vi "NCC DLL Test.vi"() -> ()   [LabVIEW 2016]
uses:
  Microscope Control/Microscope Modules/Wide Field Drift Correction/WFDC DLL and Testing/Visual Studio NCC Max Shift DLL/x64/Release/VSmaxShiftNCC.dll
panel:
  out "Time (s)":dbl
  out "Intensity Graph":dbl[][](graph)
  out "theResult":dbl[][](array[numeric])
  in  "Test Image 02":path=path "C:/Users/George Sirinakis/Documents/Microscope Control/Microscope Modules/Wide Field Drift Correction/WFDC DLL and Testing/Egg Chamber Test Data/Stack02/Color02/Color02_00001.tif"
  in  "Test Image 01":path=path "C:/Users/George Sirinakis/Documents/Microscope Control/Microscope Modules/Wide Field Drift Correction/WFDC DLL and Testing/Egg Chamber Test Data/Stack02/Color02/Color02_00007.tif"
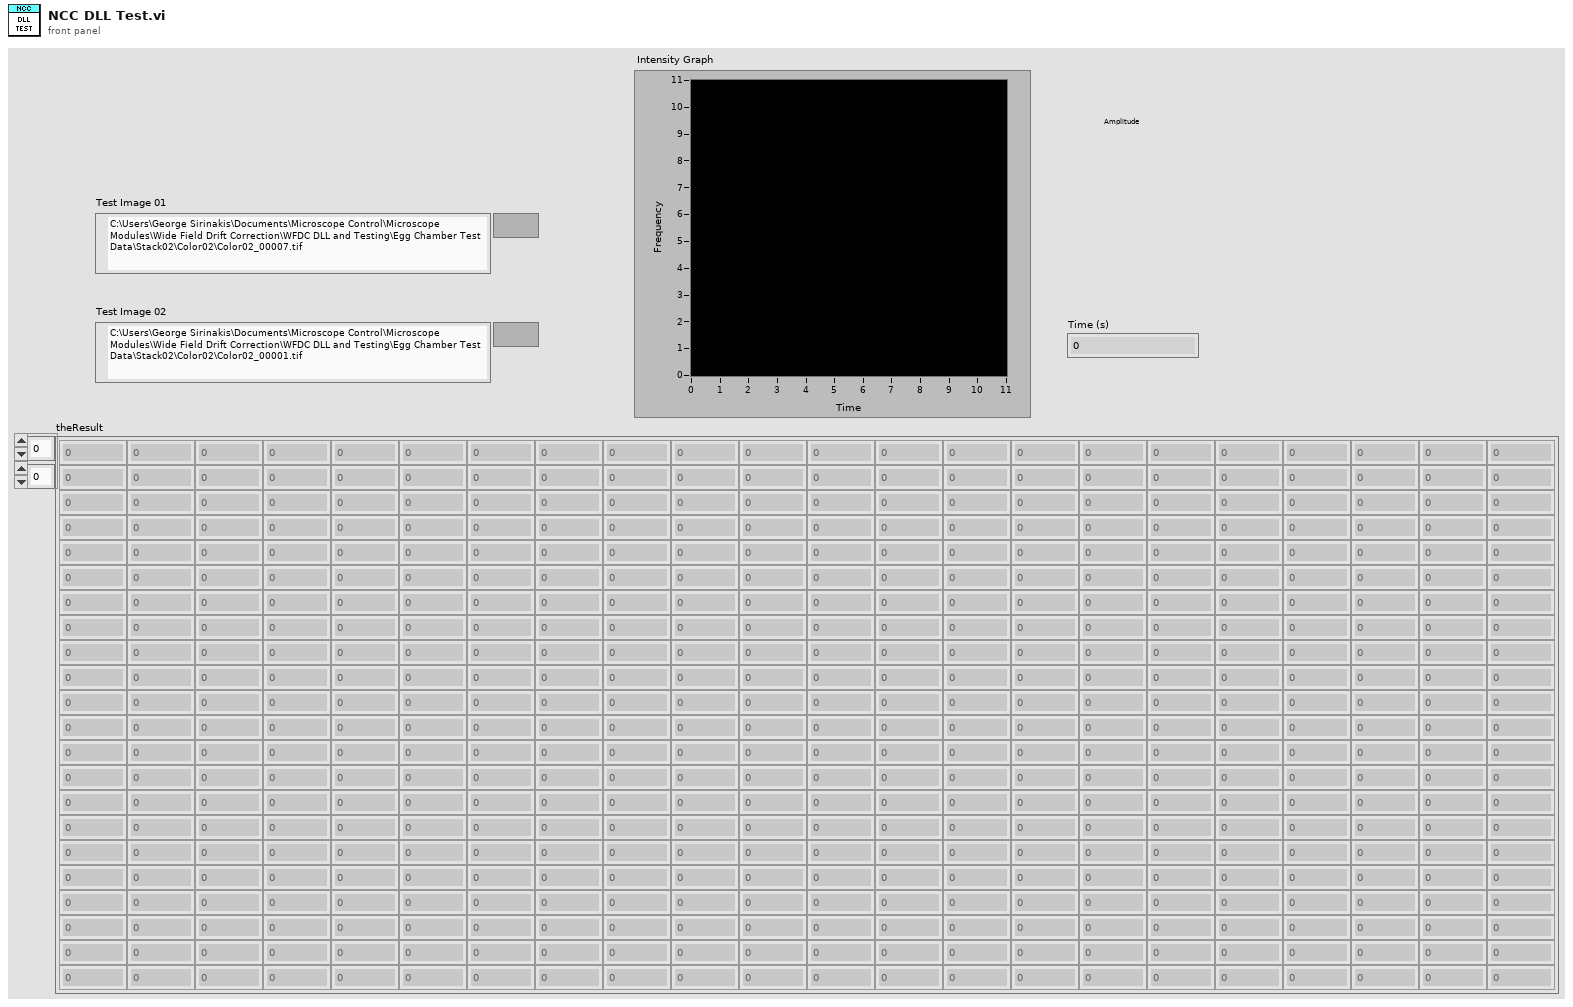
[diagram p1: front panel]
types:
  T1 = typedef "Image Type" = u32
  T2 = typedef "IMAQ Image.ctl" = refnum<image>
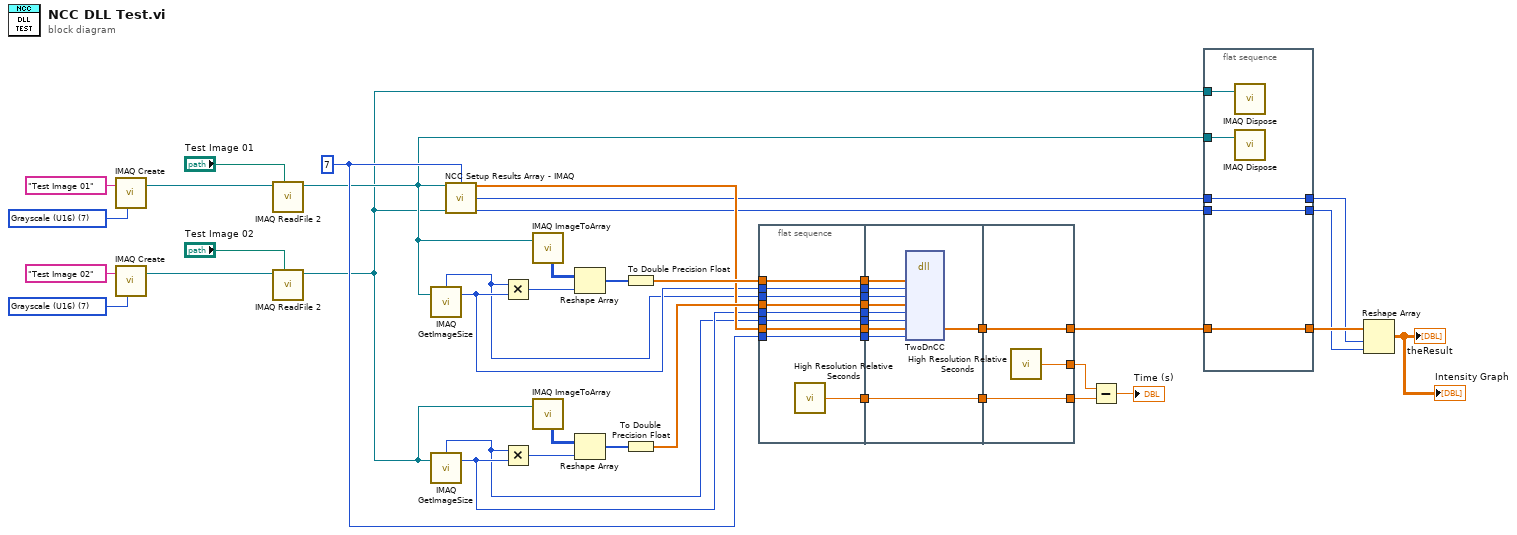
[diagram p0: block diagram]
diagram:
  w42 = T1 7 items=["Grayscale (U8)", "Grayscale (I16)", "Grayscale (SGL)", "Complex (CSG)", "RGB (U32)", "HSL (U32)", "RGB (U64)", "Grayscale (U16)"] ("Image Type")
  w43 = T1 7 items=["Grayscale (U8)", "Grayscale (I16)", "Grayscale (SGL)", "Complex (CSG)", "RGB (U32)", "HSL (U32)", "RGB (U64)", "Grayscale (U16)"] ("Image Type")
  w28 = 7 ("Half Shift")
  n1 = call "IMAQ Create"("Image Name"="Test Image 01", "Image Type"=w43) -> ("New Image"=w41:T2)  [unwired: 3 in, 1 out]
  n2 = call "IMAQ Create"("Image Name"="Test Image 02", "Image Type"=w42) -> ("New Image"=w40:T2)  [unwired: 3 in, 1 out]
  n3 = call "IMAQ ReadFile 2"("File Path"="Test Image 01", "Image"=w41) -> ("Image Out"=w22:T2)  [unwired: 5 in, 4 out]
  n4 = call "IMAQ ReadFile 2"("File Path"="Test Image 02", "Image"=w40) -> ("Image Out"=w21:T2)  [unwired: 5 in, 4 out]
  n5 = call "IMAQ GetImageSize"("Image"=w22) -> ("Y Resolution"=w25:i32, "X Resolution"=w24:i32)  [unwired: 3 in, 1 out]
  n6 = call "IMAQ GetImageSize"("Image"=w21) -> ("Y Resolution"=w27:i32, "X Resolution"=w26:i32)  [unwired: 3 in, 1 out]
  n7 = call "NCC Setup Results Array - IMAQ.vi"("Image Ref 01"=w22, "Half Shift"=w28, "Image Ref 02"=w21) -> ("NCC Results Array"=w29:dbl[], "Result Rows"=w20:i32, "Result Columns"=w19:i32)  [unwired: 10 in]
  n8 = Multiply(x=w24, y=w25) -> (x*y=w35:i32)
  n9 = Multiply(x=w26, y=w27) -> (x*y=w36:i32)
  n10 = call "IMAQ ImageToArray"("Image"=w22) -> ("Image Pixels (U16)"=w34:u16[][])  [unwired: 3 in, 4 out]
  n11 = call "IMAQ ImageToArray"("Image"=w21) -> ("Image Pixels (U16)"=w37:u16[][])  [unwired: 3 in, 4 out]
  n12 = Reshape Array(w34, w35) -> (w33:u16[])
  n13 = Reshape Array(w37, w36) -> (w32:u16[])
  n14 = To Double Precision Float(number=w33) -> (double precision float=w31:dbl[])
  n15 = To Double Precision Float(number=w32) -> (double precision float=w30:dbl[])
  n16 = flat-sequence {
    tunnel: w24 -> [w47]
    tunnel: w25 -> [w48]
    tunnel: w26 -> [w49]
    tunnel: w27 -> [w50]
    tunnel: w28 -> [w51]
    tunnel: w29 -> [w52]
    tunnel: w30 -> [w53]
    tunnel: w31 -> [w54]
    tunnel: [w54] -> w13
    tunnel: [w53] -> w12
    tunnel: [w52] -> w11
    tunnel: [w51] -> w10
    tunnel: [w50] -> w9
    tunnel: [w49] -> w8
    tunnel: [w48] -> w7
    tunnel: [w47] -> w6
    tunnel: [w46] -> w4
    tunnel: [w56] -> w14
    tunnel: w13 -> [w64]
    tunnel: w12 -> [w63]
    tunnel: w11 -> [w62]
    tunnel: w10 -> [w61]
    tunnel: w9 -> [w60]
    tunnel: w8 -> [w59]
    tunnel: w7 -> [w58]
    tunnel: w6 -> [w57]
    tunnel: [w55] -> w5
    tunnel: w4 -> [w55]
    tunnel: [w67] -> w23
    tunnel: w14 -> [w67]
    tunnel: [w66] -> w2
    tunnel: w5 -> [w66]
    tunnel: [w65] -> w3
    frame #0 {
      n17 = call <vilib>:"High Resolution Relative Seconds.vi"() -> ("relative seconds"=w46:dbl)
    }
    frame #1 {
      n18 = dll-call lib="C:/Users/George Sirinakis/Documents/Microscope Control/Microscope Modules/Wide Field Drift Correction/WFDC DLL and Testing/Visual Studio NCC Max Shift DLL/x64/Release/VSmaxShiftNCC.dll" fn="TwoDnCC"("im01"=w64, "im01rowSize"=w58, "im01colSize"=w57, "im02"=w63, "im02rowSize"=w60, "im02ColSize"=w59, "theResult"=w62, "halfShift"=w61) -> ("theResult"=w56:dbl[])  [unwired: 11 in, 2 out]
    }
    frame #2 {
      n19 = call <vilib>:"High Resolution Relative Seconds.vi"() -> ("relative seconds"=w65:dbl)
    }
  }
  n20 = Subtract(x=w3, y=w2) -> (x-y=→"Time (s)":dbl)
  n21 = flat-sequence {
    tunnel: w23 -> [w70]
    tunnel: w22 -> [w72]
    tunnel: w21 -> [w71]
    tunnel: [w70] -> w18
    tunnel: [w69] -> w16
    tunnel: w20 -> [w69]
    tunnel: w19 -> [w68]
    tunnel: [w68] -> w17
    frame #0 {
      n22 = call "IMAQ Dispose"("Image"=w71) -> ()  [unwired: 5 in, 1 out]
      n23 = call "IMAQ Dispose"("Image"=w72) -> ()  [unwired: 5 in, 1 out]
    }
  }
  n24 = Reshape Array(w18, w16, w17) -> (→"theResult" →"Intensity Graph":dbl[][])
